vi "PrepareingForRecording_171213.vi"(9 "OutputPixmapforCalculations":u32[][](array[numeric]), 10 "TTLArray":T1(array[cluster]), 11 "TotalNumberOfSegments":i32) -> (2 "Segments(s)":dbl[](array[numeric]), 3 "Segments":bool[](array[boolean]))   [LabVIEW 2016]
uses:
  Globaltracker.vi
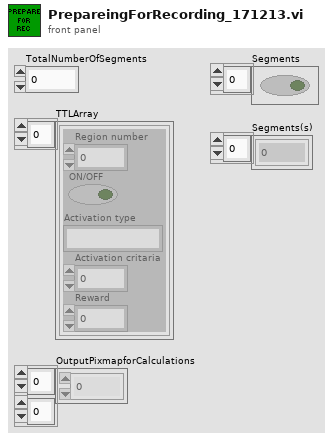
[diagram p1: front panel]
types:
  T1 = cluster{"Region number":i32, "ON/OFF":bool, "Activation type":string, "Activation critaria":i32, "Reward":i32}[]
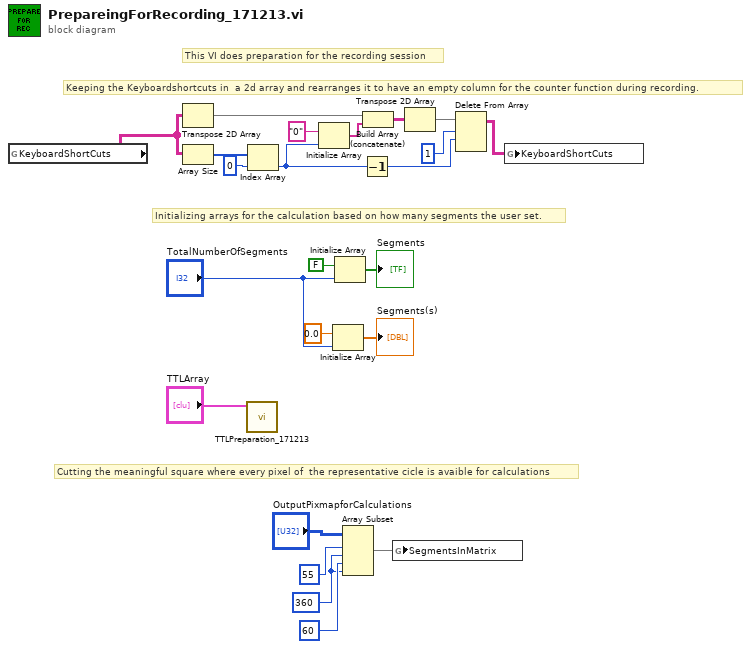
[diagram p0: block diagram]
diagram:
  w22 = 360 ("length")
  # "Keeping the Keyboardshortcuts in  a 2d array and rearranges it to have an empty column for the counter function during recording."
  # "Cutting the meaningful square where every pixel of  the representative cicle is avaible for calculations"
  # "Initializing arrays for the calculation based on how many segments the user set."
  # "This VI does preparation for the recording session"
  n1 = global read "Globaltracker.vi" "KeyboardShortCuts"() -> (w2:string[][])
  n2 = Transpose 2D Array(2D array=w2) -> (transposed array=w9:string[][])
  n3 = Array Size(array=w2) -> (size(s)=w12:i32[])
  n4 = call "TTLPreparation_171213.vi"("TTLArray"="TTLArray") -> ()  [unwired: 11 in]
  n5 = Index Array(array=w12, index=0) -> (element=w5:i32)
  n6 = Initialize Array("0", w5) -> (w8:string[])
  n7 = Initialize Array(0.0 ("element"), "TotalNumberOfSegments") -> (→"Segments(s)":dbl[])
  n8 = Initialize Array(FALSE, "TotalNumberOfSegments") -> (→"Segments":bool[])
  n9 = Array Subset(array="OutputPixmapforCalculations", index (row)=55 ("index"), length (row)=w22, index (col)=60 ("index"), length (col)=w22) -> (w19:u32[][])
  n10 = Decrement(x=w5) -> (x-1=w3:i32)
  n11 = Build Array (concatenate)(w9, w8) -> (w7:string[][])
  n12 = global write "Globaltracker.vi" "SegmentsInMatrix"(w19) -> ()
  n13 = Transpose 2D Array(2D array=w7) -> (transposed array=w6:string[][])
  n14 = Delete From Array(array=w6, length=1, index (row)=w3) -> (array with subset deleted=w1:string[][])  [unwired: 1 in, 1 out]
  n15 = global write "Globaltracker.vi" "KeyboardShortCuts"(w1) -> ()
